vi "Actor Core.vi"(8 "error in":errorcluster, 11 "State in":refnum<class "XBox Controller-Virtual.lvclass">) -> (0 "error out":errorcluster, 3 "Actor out":refnum<class "Actor.lvclass">)   [LabVIEW 2013, in "XBox Controller.lvlib" / "XBox Controller-Virtual.lvclass"]
doc: "(<B>Filename</B>: Actor Framework.lvlib:Actor.lvclass:Actor Core.vi)\n\nThis override invokes Entry.vi on the initial state, prior to calling the parent Actor Core. Adding this behavior to Actor Core (instead of an override of Pre Launch Init.vi) allows the initial state to launch a nested actor as part of its entry behavior.\n\nReceives messages to the actor, reacts to them, and initiates any error handling that may shut the actor down.\n\nDescendant classes may override this VI to append parallel tasks for the actor to complete while it handles messages. Overrides use the Call Parent Method node."
uses:
  XBox Controller-Virtual.lvclass
  <vilib>/ActorFramework/Actor/Actor.lvclass
  Robot/Virtual Systems/XBox Controller/XBox Controller Class/Joystick.ctl
  XBox Controller-Virtual.lvclass/XBox Controller-Virtual.ctl
  Robot/Virtual Systems/XBox Controller/XBox Controller Class/XBox Controller-Logical.lvclass
  Robot/Logical Systems/XBox Controller/XBox Controller Class/Xbox Controller.lvlib
panel:
  in  "Driver Joystick":T1 {"Right" scale=-1.0..1.0; "Forward" scale=-1.0..1.0}
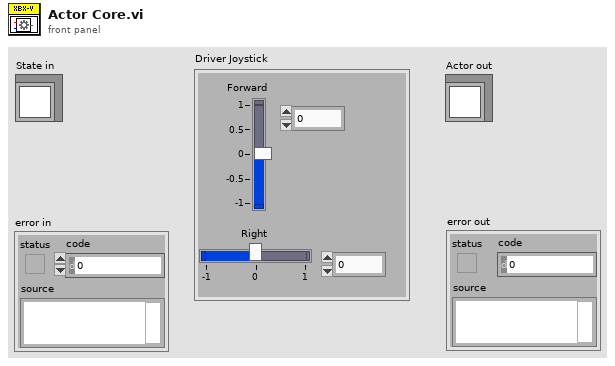
[diagram p1: front panel]
types:
  T1 = typedef "Logical Systems.lvlib/Xbox Controller.lvlib/Joystick.ctl" = cluster{"Forward":dbl, "Right":dbl}
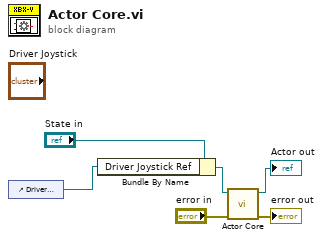
[diagram p0: block diagram]
diagram:
  n1 = control-ref of="Driver Joystick"() -> (w1:refnum<vi>)
  n2 = Bundle By Name(cluster="State in", "Driver Joystick Ref"=w1) -> (w2:refnum<class "XBox Controller-Virtual.lvclass">)
  n3 = call-parent "Actor Core.vi"("error in"="error in", "State in"=w2) -> ("error out"=→"error out":errorcluster, "Actor out"=→"Actor out":refnum<class "Actor.lvclass">)  [unwired: 8 in]
